vi "TimeToSpeedArray (SubVI).vi"(11 "Array":dbl[](array[numeric])) -> (3 "Array 2":dbl[](array[numeric]))   [LabVIEW 2017]
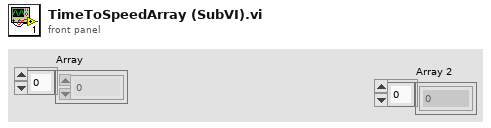
[diagram p1: front panel]
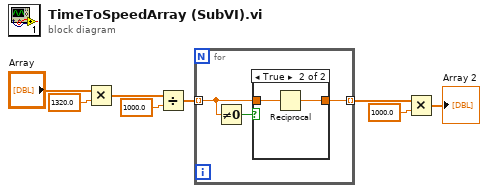
[diagram p0: block diagram]
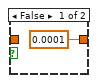
[diagram p2: hidden frame]
diagram:
  n1 = Multiply(x="Array", y=1320.0) -> (x*y=w7:dbl[])
  n2 = Divide(x=w7, y=1000.0) -> (x/y=w5:dbl[])
  n3 = for {
    tunnel: w5 -> [w11] mode=indexing
    tunnel: [w10] -> w4 mode=indexing
    n4 = Not Equal To 0?(x=w11) -> (x != 0?=w9:bool)
    n5 = case shown="True" w9 {
      tunnel: w11 -> [_ w14]
      tunnel: [0.0001 ("f") w13] -> w10
      frame False {
      }
      frame True {
        n6 = Reciprocal(x=w14) -> (1/x=w13:dbl)
      }
    }
  }
  n7 = Multiply(x=w4, y=1000.0) -> (x*y=→"Array 2":dbl[])
